vi "USB2XXX_LIN_SlaveTest.vi"() -> ()   [LabVIEW 2010]
uses:
  PublicFiles/USB2XXX.dll
panel:
  in  "pConfig":T1
  in  "pLINMsgBuffer":T2
  out "pLINMsg":T2
  in  "stop":bool
  in  "Channel Index":u8(ring) items=["CH0"]
  in  "Device Index":i32(ring) items=["0", "1", "2", "3", "4", "5"]
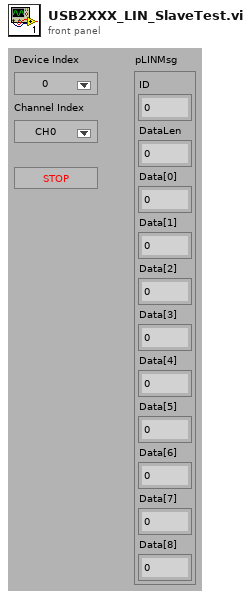
[diagram p1: front panel]
types:
  T1 = cluster{"BaudRate":u32, "CheckMode":u8, "MasterMode":u8, "BreakBits":u8}
  T2 = cluster{"ID":u8, "DataLen":u8, "Data[0]":u8, "Data[1]":u8, "Data[2]":u8, "Data[3]":u8, "Data[4]":u8, "Data[5]":u8, "Data[6]":u8, "Data[7]":u8, "Data[8]":u8}
  T3 = cluster{"ID":u8, "DataLen":u8, "Data[0]":u8, "Data[1]":u8, "Data[2]":u8, "Data[3]":u8, "Data[4]":u8, "Data[5]":u8, "Data[6]":u8, "Data[7]":u8, "Data[8]":u8}[]
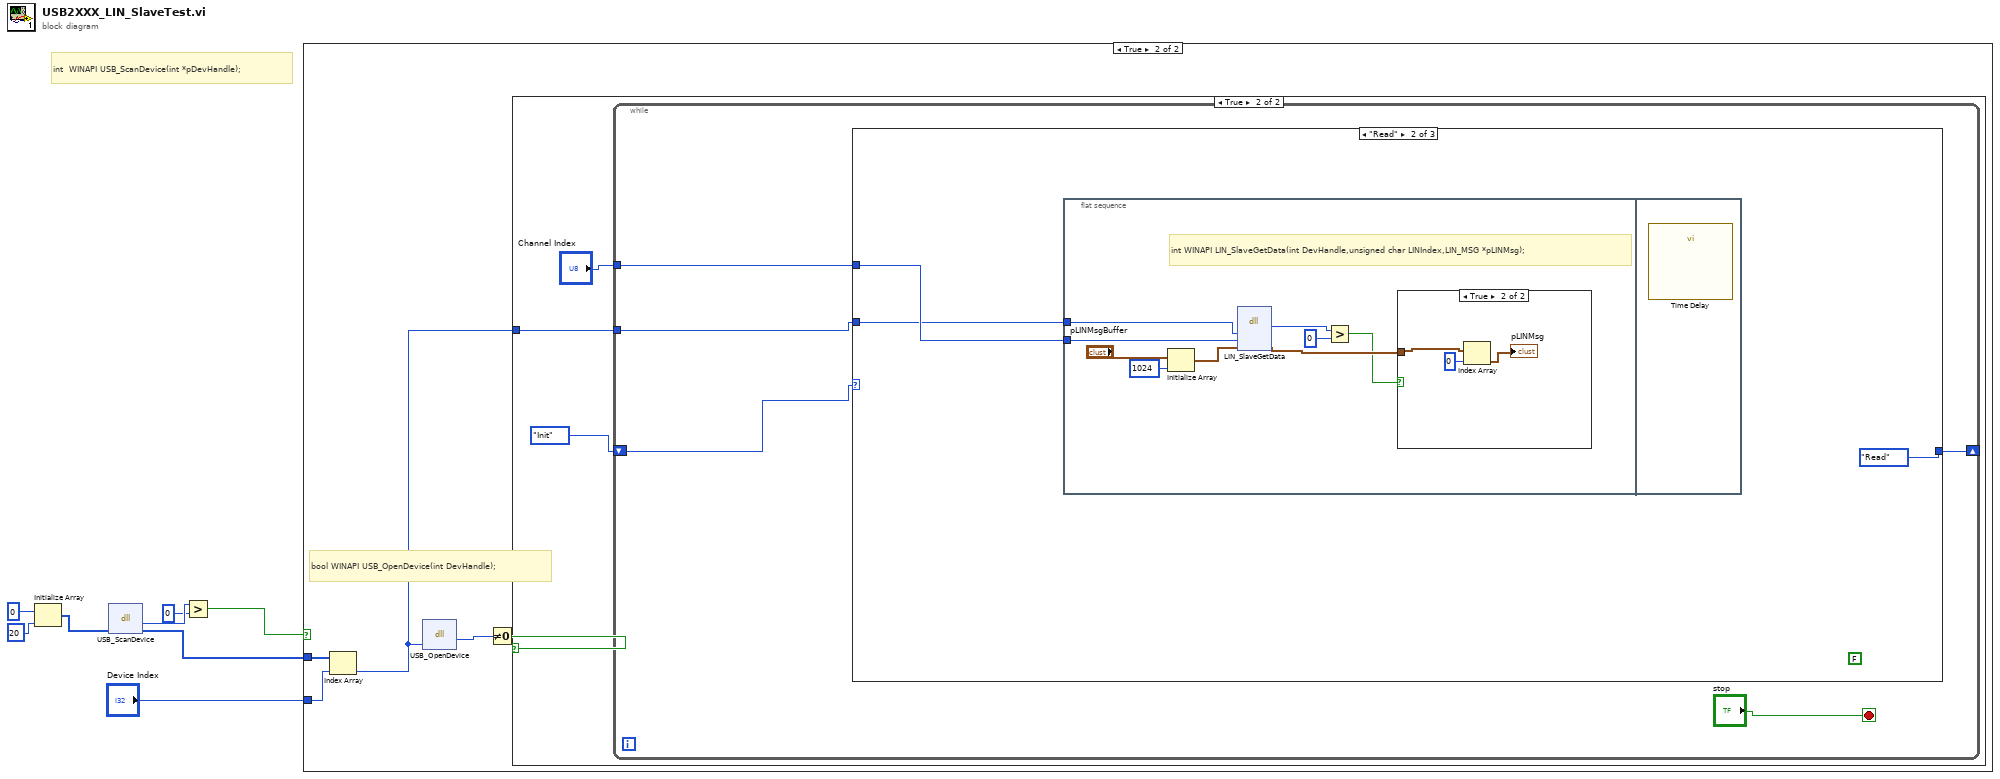
[diagram p0: block diagram]
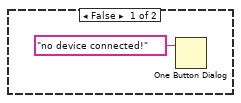
[diagram p2: hidden frame]
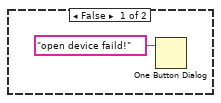
[diagram p3: hidden frame]
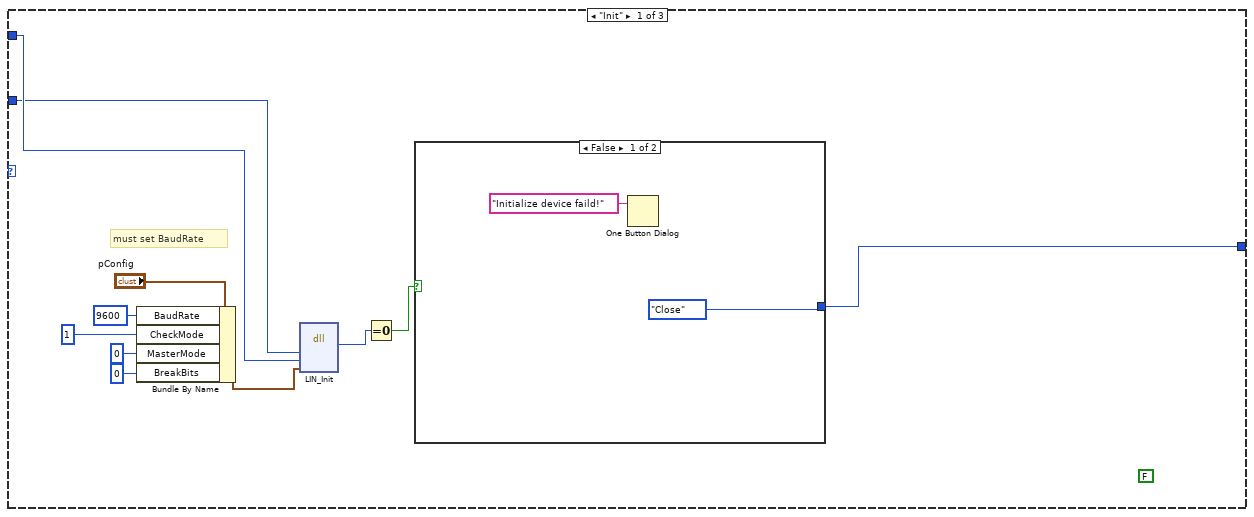
[diagram p4: hidden frame]
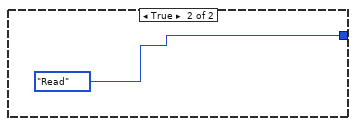
[diagram p5: hidden frame]
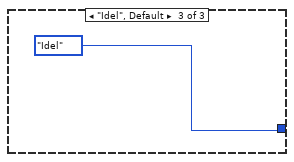
[diagram p7: hidden frame]
diagram:
  # "int  WINAPI USB_ScanDevice(int *pDevHandle);"
  n1 = Initialize Array(0, 20 ("dimension size")) -> (w6:i32[])
  n2 = dll-call lib="E:/OtherWork/STM32/USB2XXX_Example/trunk/Labview/PublicFiles/USB2XXX.*" fn="USB_ScanDevice"("pDevHandle"=w6) -> (w5:i32, "pDevHandle"=w2:i32[])  [unwired: 3 in, 2 out]
  n3 = Greater?(x=w5, y=0) -> (0:w3:bool)
  n4 = case shown="True" w3 {
    tunnel: w2 -> [_ w14]
    tunnel: "Device Index" -> [_ w13]
    frame False {
      n5 = One Button Dialog(message="no device connected!") -> ()  [unwired: 1 in, 1 out]
    }
    frame True {
      # "bool WINAPI USB_OpenDevice(int DevHandle);"
      n6 = Index Array(array=w14, index=w13) -> (element=w10:i32)
      n7 = dll-call lib="E:/OtherWork/STM32/USB2XXX_Example/trunk/Labview/PublicFiles/USB2XXX.*" fn="USB_OpenDevice"("DevHandle"=w10) -> (w12:u8)  [unwired: 4 in, 2 out]
      n8 = Not Equal To 0?(x=w12) -> (x != 0?=w11:bool)
      n9 = case shown="True" w11 {
        tunnel: w10 -> [_ w17]
        frame False {
          n10 = One Button Dialog(message="open device faild!") -> ()  [unwired: 1 in, 1 out]
        }
        frame True {
          n11 = while {
            shift-right: [w22] -> _
            shift-left: enum16{"Init", "Write", "Read", "Idel", "Close"}."Init" ("Enum") -> [w19]
            tunnel: w17 -> [w21]
            tunnel: "Channel Index" -> [w20]
            stop <- "stop" stop-if-true
            n12 = case shown="\"Read\"" w19 {
              tunnel: [w24 enum16{"Init", "Write", "Read", "Idel", "Close"}."Read" ("Enum") enum16{"Init", "Write", "Read", "Idel", "Close"}."Idel" ("Enum")] -> w22
              tunnel: w21 -> [w25 w38 _]
              tunnel: w20 -> [w26 w39 _]
              frame "Init" {
                (unwired) FALSE
                # "must set BaudRate"
                n13 = Bundle By Name(cluster="pConfig", "BaudRate"=u32 9600, "CheckMode"=u16 1 ("OwnAddr"), "MasterMode"=u8 0 ("Master"), "BreakBits"=u8 0 ("AddrBits")) -> (w29:T1)
                n14 = dll-call lib="E:/OtherWork/STM32/USB2XXX_Example/trunk/Labview/PublicFiles/USB2XXX.*" fn="LIN_Init"("DevHandle"=w25, "LINIndex"=w26, "pConfig"=w29) -> (w28:i32)  [unwired: 6 in, 2 out]
                n15 = Equal To 0?(x=w28) -> (x = 0?=w31:bool)
                n16 = case shown="False" w31 {
                  tunnel: [enum16{"Init", "Write", "Read", "Idel", "Close"}."Close" ("Enum") enum16{"Init", "Write", "Read", "Idel", "Close"}."Read" ("Enum")] -> w24
                  frame False {
                    n17 = One Button Dialog(message="Initialize device faild!") -> ()  [unwired: 1 in, 1 out]
                  }
                  frame True {
                  }
                }
              }
              frame "Read" {
                (unwired) FALSE
                n18 = flat-sequence {
                  tunnel: w39 -> [w42]
                  tunnel: w38 -> [w41]
                  frame #0 {
                    # "int WINAPI LIN_SlaveGetData(int DevHandle,unsigned char LINIndex,LIN_MSG *pLINMsg);"
                    n19 = Initialize Array("pLINMsgBuffer", 1024 ("dimension size")) -> (w45:T3)
                    n20 = dll-call lib="E:/OtherWork/STM32/USB2XXX_Example/trunk/Labview/PublicFiles/USB2XXX.*" fn="LIN_SlaveGetData"("DevHandle"=w41, "LINIndex"=w42, "pLINMsg"=w45) -> ("return type"=w46:i32, "pLINMsg"=w49:T3)  [unwired: 5 in, 2 out]
                    n21 = Greater?(x=w46, y=0) -> (0:w48:bool)
                    n22 = case shown="True" w48 {
                      tunnel: w49 -> [_ w50]
                      frame False {
                      }
                      frame True {
                        n23 = Index Array(array=w50, index=0) -> (element=→"pLINMsg":T2)
                      }
                    }
                  }
                  frame #1 {
                    n24 = call "Time Delay"() -> ()  [unwired: 11 in, 1 out]
                  }
                }
              }
              frame "Idel", Default {
              }
            }
          }
        }
      }
    }
  }
